vi "LabVIEW Basics #3 - Servo Sweep.vi"() -> ()   [LabVIEW 2019]
uses:
  <vilib>/MakerHub/LINX/Public/Utilities/Open Serial.vi
  <vilib>/MakerHub/LINX/Public/Sensors/Motion/Servo/Servo Open One Channel.vi
  <vilib>/MakerHub/LINX/Public/Sensors/Motion/Servo/Servo Set Pulse Width One Channel.vi
  <vilib>/MakerHub/LINX/Public/Sensors/Motion/Servo/Servo Close One Channel.vi
  <vilib>/MakerHub/LINX/LMH-LINX.lvlib
  <vilib>/MakerHub/LINX/Public/Sensors/Motion/Servo/Servo.lvlib
panel:
  in  "Period":u32(slide)=100 caption="Period (ms)" max=1000 step=50 scale=0.0..1000.0
  out "Device Name":string
  in  "Stop":bool
  out "Angle (°)":dbl
  out "Pulse Width (uS)":dbl
  # "General Controls"
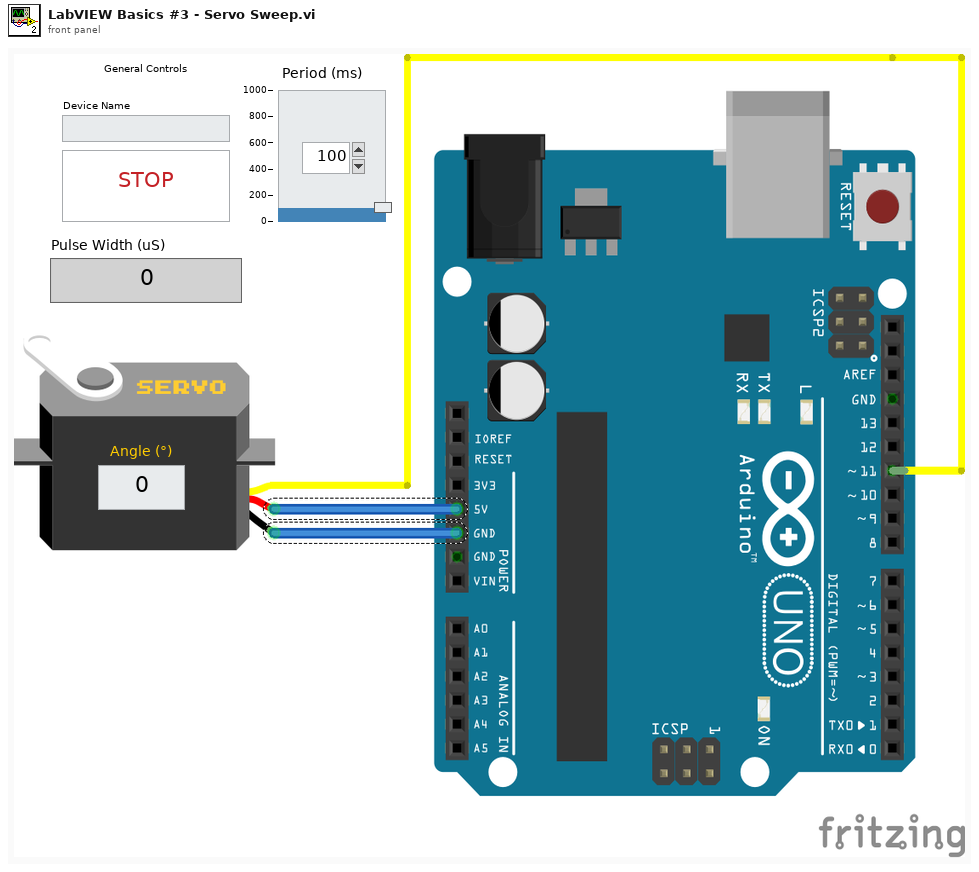
[diagram p1: front panel]
types:
  T1 = typedef "LMH-LINX.lvlib/LINX Ref.ctl" = cluster{"IO":T2, "Interface":T3, "LINX Device Config":T4}
  T2 = typedef "LMH-LINX.lvlib/Platform.ctl" = enum16{"Remote", "Local"}
  T3 = typedef "LMH-LINX.lvlib/Interface.ctl" = enum16{"Serial", "TCP"}
  T4 = typedef "LMH-LINX.lvlib/Device.lvlib/LINX Device Config.ctl" = cluster{"Interface":T3, "COM Port":refnum<visa-resource-name>, "TCP Configuration":T5, "Device Family":u8, "Device ID":u8, "Device Name":string, "TCP Ref":refnum<k5>, "Channels":T6}
  T5 = typedef "LMH-LINX.lvlib/Device.lvlib/TCP Config.ctl" = cluster{"IP Address":string, "Port":u16}
  T6 = typedef "LMH-LINX.lvlib/Channels.ctl" = cluster{"DI":u8[], "DO":u8[], "AI":u8[], "AO":u8[], "PWM":u8[], "QE":u8[], "UART":u8[], "I2C 2":u8[], "SPI":u8[], "CAN":u8[], "Servo":u8[], "AI Ref (V)":dbl, "AI Resolution (Bits)":u8, "AO Ref (V)":dbl, "AO Resolution (Bits)":u8}
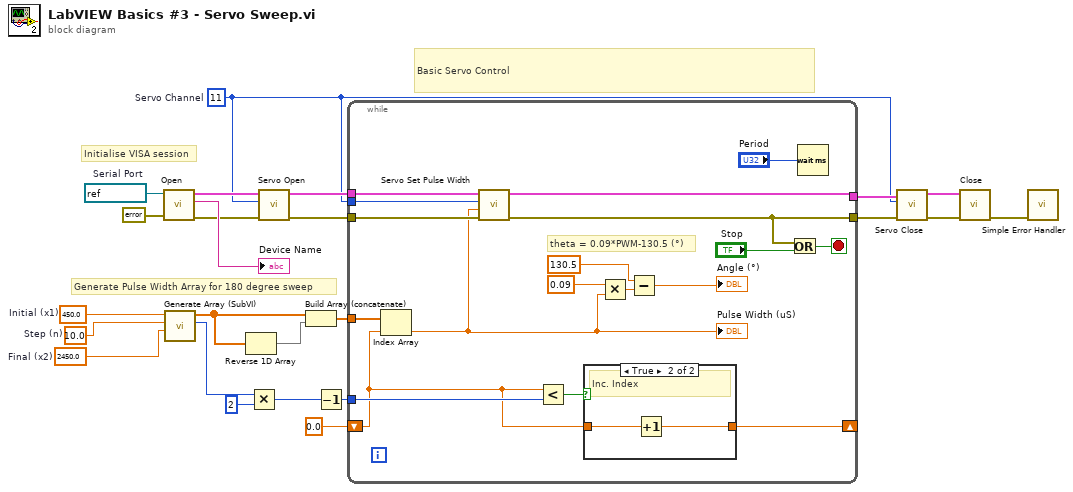
[diagram p0: block diagram]
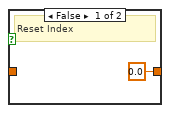
[diagram p2: hidden frame]
diagram:
  w9 = 2450.0  # Final (x2)
  w8 = 10.0  # Step (n)
  w7 = 450.0  # Initial (x1)
  w12 = u8 11  # Servo Channel
  w24 = refnum<visa-resource-name> "COM6"  # Serial Port
  # "Generate Pulse Width Array for 180 degree sweep"
  # "Initialise VISA session"
  # "Basic Servo Control"
  n1 = call-poly <vilib>:"Open.vi"("Error In"=errorcluster {"status"=FALSE, "code"=0, "source"=""}, "Serial Port"=w24) -> ("Error Out"=w17:errorcluster, "Device Name"=→"Device Name":string, "LINX Resource"=w18:T1)  [unwired: 7 in]
  n2 = call "Generate Array (SubVI).vi"("Final"=w9, "Step"=w8, "Initial"=w7) -> ("Array size"=w2:i32, "Array out"=w5:dbl[])  [unwired: 6 in, 1 out]
  n3 = Reverse 1D Array(array=w5) -> (reversed array=w4:dbl[])
  n4 = Multiply(x=w2, y=2) -> (x*y=w3:i32)
  n5 = call-poly <vilib>:"Servo Open.vi"("Error In"=w17, "Servo Channel"=w12, "LINX Resource"=w18) -> ("Error Out"=w15:errorcluster, "LINX Resource"=w16:T1)  [unwired: 7 in]
  n6 = Build Array (concatenate)(w5, w4) -> (w6:dbl[])
  n7 = Decrement(x=w3) -> (x-1=w10:i32)
  n8 = while {
    tunnel: [w25] -> w20
    tunnel: [w34] -> w19
    tunnel: w16 -> [w40]
    tunnel: w15 -> [w39]
    tunnel: w12 -> [w33]
    tunnel: w6 -> [w32]
    shift-right: [w31] -> _
    shift-left: 0.0 -> [w27]
    tunnel: w10 -> [w29]
    stop <- w41 stop-if-true
    # "theta = 0.09*PWM-130.5 (°)"
    n9 = Index Array(array=w32, index=w27) -> (element=w28:dbl)
    "Pulse Width (uS)" <- w28
    n10 = call-poly <vilib>:"Servo Set Pulse Width.vi"("Error In"=w39, "Pulse Width (uS)"=w28, "Servo Channel"=w33, "LINX Resource"=w40) -> ("Error Out"=w34:errorcluster, "LINX Resource"=w25:T1)  [unwired: 6 in]
    n11 = Less?(x=w27, y=w29) -> (x < y?=w26:bool)
    n12 = case shown="True" w26 {
      tunnel: [0.0 w45] -> w31
      tunnel: w27 -> [_ w44]
      frame False {
        # "Reset Index"
      }
      frame True {
        # "Inc. Index"
        n13 = Increment(x=w44) -> (x+1=w45:dbl)
      }
    }
    n14 = Multiply(x=0.09, y=w28) -> (x*y=w36:dbl)
    n15 = Subtract(x=130.5, y=w36) -> (x-y=→"Angle (°)":dbl)
    n16 = Or(x=w34, y="Stop") -> (x .or. y?=w41:bool)
    n17 = Wait (ms)(milliseconds to wait="Period") -> ()  [unwired: 1 out]
  }
  n18 = call-poly <vilib>:"Servo Close.vi"("Error In"=w19, "Servo Channel"=w12, "LINX Resource"=w20) -> ("Error Out"=w14:errorcluster, "LINX Resource"=w13:T1)  [unwired: 7 in]
  n19 = call <vilib>:"Close.vi"("Error In"=w14, "LINX Resource"=w13) -> ("Error Out"=w21:errorcluster)  [unwired: 9 in]
  n20 = call <vilib>:"Simple Error Handler.vi"("error in (no error)"=w21) -> ()  [unwired: 4 in, 5 out]
